vi "Initialize Protection Frames Incoming.vi"(8 "error in (no error)":errorcluster, 10 "Frames":T2[](array[typedef]) {"Protection Configurations"."CRC Channels"."Data Type" items=["Signed", "Unsigned", "IEEE Float"]}, 11 "PCL (usec)":u32) -> (0 "error out":errorcluster, 1 "Frame Values":T1, 2 "RT Frames":T9[](array[typedef]) {"Protection Configurations"."CRC Channels"."Data Type" items=["Signed", "Unsigned", "IEEE Float"]})   [LabVIEW 2023, in "Protection and Counter Support Engine.lvlib"]
uses:
  Protection and Counter Support Engine.lvlib
  Types/RT Frame Settings.ctl
  Shared/Types/Exported Frame Type.ctl
  Types/RT Protection Configuration.ctl
  Shared/Types/Protection Type.ctl
  Shared/Types/XNET Signal Configuration.ctl
  Shared/Types/Exported Counter Settings.ctl
  Shared/Types/Exported Event Trigger Type.ctl
  Shared/Types/Exported Frame Settings.ctl
  Shared/Types/Exported Protection Settings.ctl
  Types/RT Frame Incoming Values.ctl
  <vilib>/xnet/xnet.llb/XNET Create Session (Conversion).vi
  Shared/Protection and Counter Support Shared.lvlib
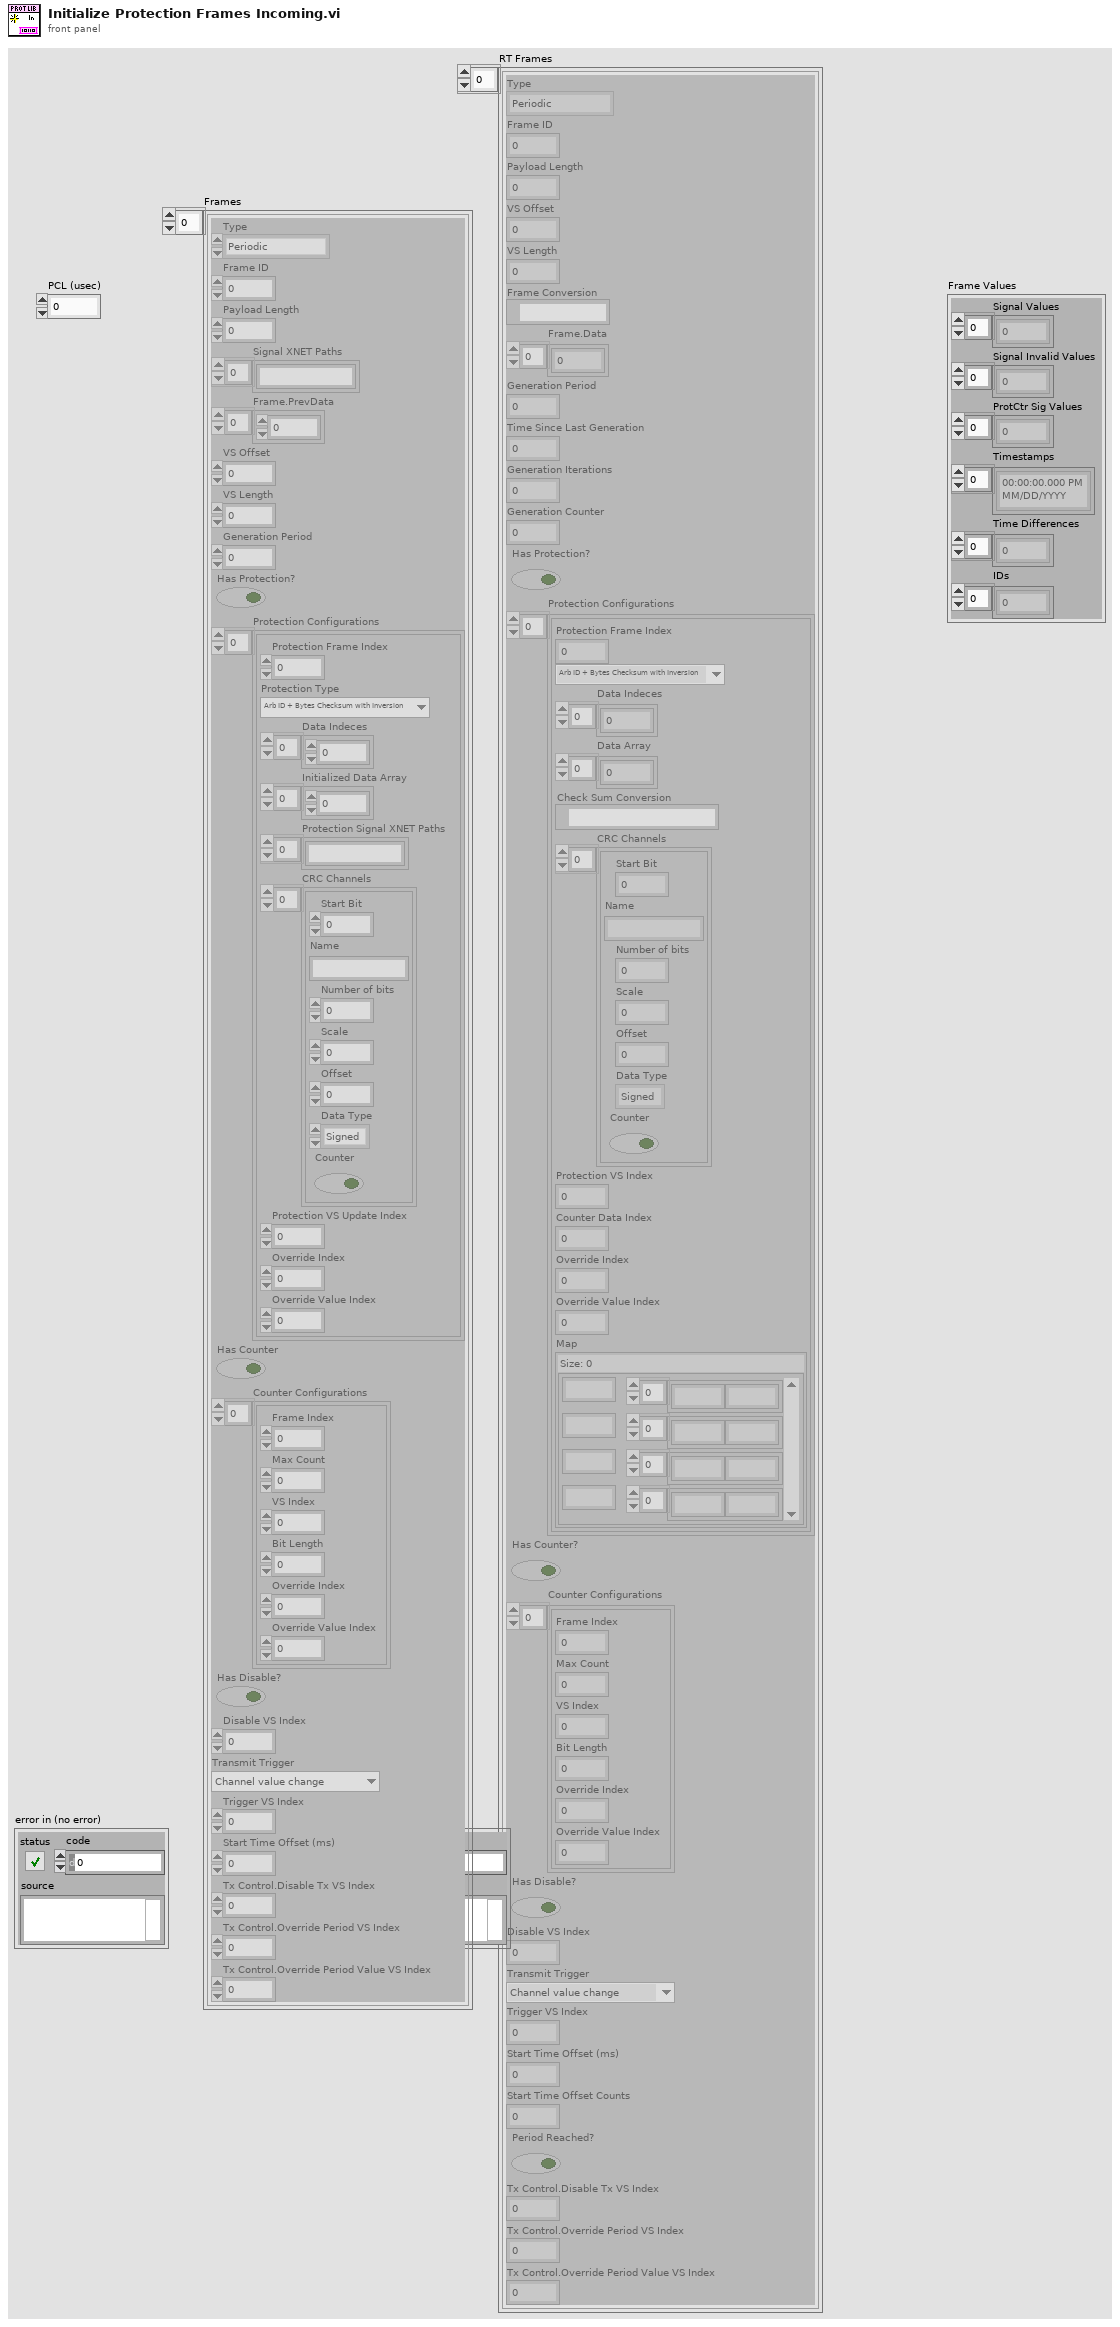
[diagram p1: front panel]
types:
  T1 = typedef "Protection and Counter Support Engine.lvlib/RT Frame Incoming Values.ctl" = cluster{"Signal Values":dbl[], "Signal Invalid Values":dbl[], "ProtCtr Sig Values":dbl[], "Timestamps":timestamp[], "Time Differences":dbl[], "IDs":u32[]}
  T2 = typedef "Protection and Counter Support Shared.lvlib/Exported Frame Settings.ctl" = cluster{"Type":T3, "Frame ID":u32, "Payload Length":u32, "Signal XNET Paths":string[], "Frame.PrevData":dbl[], "VS Offset":i32, "VS Length":i32, "Generation Period":u32, "Has Protection?":bool, "Protection Configurations":T4[], "Has Counter":bool, "Counter Configurations":T7[], "Has Disable?":bool, "Disable VS Index":i32, "Transmit Trigger":T8, "Trigger VS Index":i32, "Start Time Offset (ms)":u32, "Tx Control.Disable Tx VS Index":i32, "Tx Control.Override Period VS Index":i32, "Tx Control.Override Period Value VS Index":i32}
  T3 = typedef "Protection and Counter Support Shared.lvlib/Exported Frame Type.ctl" = enum16{"Periodic", "Event", "Periodic/Event"}
  T4 = typedef "Protection and Counter Support Shared.lvlib/Exported Protection Settings.ctl" = cluster{"Protection Frame Index":i32, "Protection Type":T5, "Data Indeces":i32[], "Initialized Data Array":dbl[], "Protection Signal XNET Paths":string[], "CRC Channels":T6[], "Protection VS Update Index":i32, "Override Index":i32, "Override Value Index":i32}
  T5 = typedef "Protection and Counter Support Shared.lvlib/Protection Type.ctl" = enum16{"Arb ID + Bytes Checksum with Inversion", "Arb ID + Bytes CRC with Inversion", "Reversed Raw Signal Checksum with Inversion", "Concatenated Two's Compliment", "LP_CRC8", "LP_Checksum", "LP_CRC8_MRS"}
  T6 = typedef "Protection and Counter Support Shared.lvlib/XNET Signal Configuration.ctl" = cluster{"Start Bit":i32, "Name":string, "Number of bits":i32, "Scale":dbl, "Offset":dbl, "Data Type":u32, "Counter":bool}
  T7 = typedef "Protection and Counter Support Shared.lvlib/Exported Counter Settings.ctl" = cluster{"Frame Index":i32, "Max Count":dbl, "VS Index":i32, "Bit Length":i64, "Override Index":i32, "Override Value Index":i32}
  T8 = typedef "Protection and Counter Support Shared.lvlib/Exported Event Trigger Type.ctl" = enum16{"Channel value change", "Trigger channel (not zero)", "Channel value change or trigger channel (not zero)", "Trigger channel (any value change)", "Channel value change or trigger channel (any value change)"}
  T9 = typedef "Protection and Counter Support Engine.lvlib/RT Frame Settings.ctl" = cluster{"Type":T3, "Frame ID":u32, "Payload Length":u32, "VS Offset":i32, "VS Length":i32, "Frame Conversion":refnum<k21>, "Frame.Data":dbl[], "Generation Period":u32, "Time Since Last Generation":u32, "Generation Iterations":u32, "Generation Counter":u32, "Has Protection?":bool, "Protection Configurations":T10[], "Has Counter?":bool, "Counter Configurations":T7[], "Has Disable?":bool, "Disable VS Index":i32, "Transmit Trigger":T8, "Trigger VS Index":i32, "Start Time Offset (ms)":u32, "Start Time Offset Counts":u32, "Period Reached?":bool, "Tx Control.Disable Tx VS Index":i32, "Tx Control.Override Period VS Index":i32, "Tx Control.Override Period Value VS Index":i32}
  T10 = typedef "Protection and Counter Support Engine.lvlib/RT Protection Configuration.ctl" = cluster{"Protection Frame Index":i32, "Protection Type":T5, "Data Indeces":i32[], "Data Array":dbl[], "Check Sum Conversion":refnum<k21>, "CRC Channels":T6[], "Protection VS Index":i32, "Counter Data Index":i32, "Override Index":i32, "Override Value Index":i32, "Map":map{i32, u8[]}}
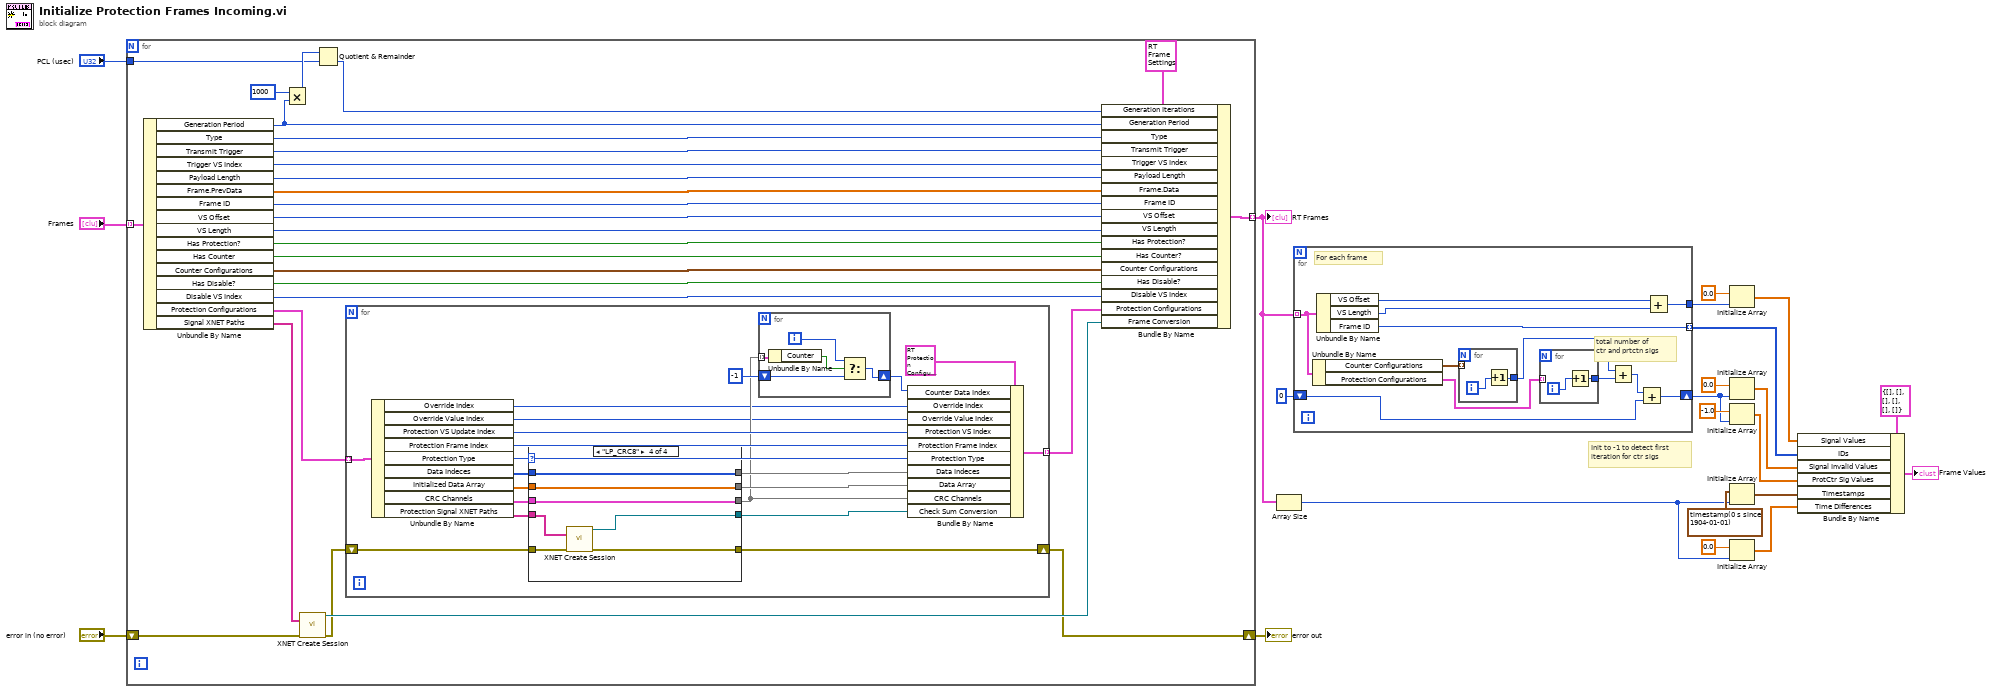
[diagram p0: block diagram]
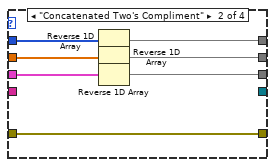
[diagram p3: hidden frame]
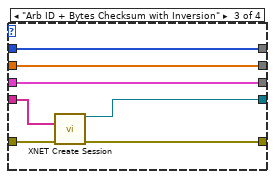
[diagram p4: hidden frame]
diagram:
  # "Init to -1 to detect first \niteration for ctr sigs"
  n1 = for {
    shift-right: [w35] -> w20
    shift-left: "error in (no error)" -> [w48]
    tunnel: "Frames" -> [w50] mode=indexing
    tunnel: [w34] -> w1 mode=indexing
    tunnel: "PCL (usec)" -> [w29]
    n2 = Unbundle By Name(w50) -> ("Generation Period"=w28:u32, "Type"=w23:T3, "Transmit Trigger"=w24:T8, "Trigger VS Index"=w25:i32, "Payload Length"=w26:u32, "Frame.PrevData"=w32:dbl[], "Frame ID"=w46:u32, "VS Offset"=w45:i32, "VS Length"=w44:i32, "Has Protection?"=w43:bool, "Has Counter"=w42:bool, "Counter Configurations"=w41:T7[], "Has Disable?"=w40:bool, "Disable VS Index"=w39:i32, "Protection Configurations"=w38:T4[], "Signal XNET Paths"=w49:string[])
    n3 = Multiply(x=u32 1000, y=w28) -> (x*y=w30:u32)
    n4 = call-poly <vilib>:"XNET Create Session.vi"("signal list"=w49, "error in (no error)"=w48) -> ("session out"=w47:refnum<k21>, "error out"=w36:errorcluster)  [unwired: 12 out]
    n5 = Quotient & Remainder(x=w30, y=w29) -> (floor(x/y)=w27:u32)  [unwired: 1 out]
    n6 = for {
      tunnel: w38 -> [w70] mode=indexing
      tunnel: [w65] -> w37 mode=indexing
      shift-right: [w63] -> w35
      shift-left: w36 -> [w64]
      n7 = Unbundle By Name(w70) -> ("Override Index"=w52:i32, "Override Value Index"=w51:i32, "Protection VS Update Index"=w54:i32, "Protection Frame Index"=w68:i32, "Protection Type"=w60:T5, "Data Indeces"=w55:i32[], "Initialized Data Array"=w57:dbl[], "CRC Channels"=w59:T6[], "Protection Signal XNET Paths"=w67:string[])
      n8 = case shown="\"LP_CRC8\"" w60 {
        tunnel: w67 -> [_ _ w88 w95]
        tunnel: [_ _ w87 w94] -> w66
        tunnel: w64 -> [w74 w81 w86 w93]
        tunnel: [w74 w81 w85 w92] -> w63
        tunnel: [w73 w77 w84 w91] -> w53
        tunnel: w59 -> [w73 w80 w84 w91]
        tunnel: [w72 w76 w83 w90] -> w58
        tunnel: w57 -> [w72 w79 w83 w90]
        tunnel: [w71 w75 w82 w89] -> w56
        tunnel: w55 -> [w71 w78 w82 w89]
        frame Default {
        }
        frame "Concatenated Two's Compliment" {
          n9 = Reverse 1D Array(array=w78) -> (reversed array=w75:i32[])
          n10 = Reverse 1D Array(array=w79) -> (reversed array=w76:dbl[])
          n11 = Reverse 1D Array(array=w80) -> (reversed array=w77:T6[])
        }
        frame "Arb ID + Bytes Checksum with Inversion" {
          n12 = call-poly <vilib>:"XNET Create Session.vi"("signal list"=w88, "error in (no error)"=w86) -> ("session out"=w87:refnum<k21>, "error out"=w85:errorcluster)  [unwired: 12 out]
        }
        frame "LP_CRC8" {
          n13 = call-poly <vilib>:"XNET Create Session.vi"("signal list"=w95, "error in (no error)"=w93) -> ("session out"=w94:refnum<k21>, "error out"=w92:errorcluster)  [unwired: 12 out]
        }
      }
      n14 = for {
        tunnel: w53 -> [w100] mode=indexing
        shift-right: [w96] -> w61
        shift-left: -1 -> [w98]
        i -> [w97]
        n15 = Unbundle By Name(w100) -> ("Counter"=w99:bool)
        n16 = Select(t=w97, s=w99, f=w98) -> (s? t:f=w96:i32)
      }
      n17 = Bundle By Name(cluster=T10 {"Protection Frame Index"=0, "Protection Type"=enum."Arb ID + Bytes Checksum with Inversion", "Data Indeces"=[], "Data Array"=[], "Check Sum Conversion"="", "CRC Channels"=[], "Protection VS Index"=0, "Counter Data Index"=0, "Override Index"=0, "Override Value Index"=0, "Map"={}} ("Cluster"), "Counter Data Index"=w61, "Override Index"=w52, "Override Value Index"=w51, "Protection VS Index"=w54, "Protection Frame Index"=w68, "Protection Type"=w60, "Data Indeces"=w56, "Data Array"=w58, "CRC Channels"=w53, "Check Sum Conversion"=w66) -> (w65:T10)
    }
    n18 = Bundle By Name(cluster=T9 {"Type"=enum."Periodic", "Frame ID"=0, "Payload Length"=0, "VS Offset"=0, "VS Length"=0, "Frame Conversion"="", "Frame.Data"=[], "Generation Period"=0, "Time Since Last Generation"=0, "Generation Iterations"=0, "Generation Counter"=0, "Has Protection?"=FALSE, "Protection Configurations"=[], "Has Counter?"=FALSE, "Counter Configurations"=[], "Has Disable?"=FALSE, "Disable VS Index"=0, "Transmit Trigger"=enum."Channel value change", "Trigger VS Index"=0, "Start Time Offset (ms)"=0, "Start Time Offset Counts"=0, "Period Reached?"=FALSE, "Tx Control.Disable Tx VS Index"=0, "Tx Control.Override Period VS Index"=0, "Tx Control.Override Period Value VS Index"=0} ("Frame Settings"), "Generation Iterations"=w27, "Generation Period"=w28, "Type"=w23, "Transmit Trigger"=w24, "Trigger VS Index"=w25, "Payload Length"=w26, "Frame.Data"=w32, "Frame ID"=w46, "VS Offset"=w45, "VS Length"=w44, "Has Protection?"=w43, "Has Counter?"=w42, "Counter Configurations"=w41, "Has Disable?"=w40, "Disable VS Index"=w39, "Protection Configurations"=w37, "Frame Conversion"=w47) -> (w34:T9)
  }
  "RT Frames" <- w1
  "error out" <- w20
  n19 = Array Size(array=w1) -> (size(s)=w6:i32)
  n20 = for {
    tunnel: w1 -> [w108] mode=indexing
    tunnel: [w112] -> w18 mode=indexing
    tunnel: [w109] -> w16
    shift-right: [w102] -> w12
    shift-left: 0 -> [w101]
    # "total number of\nctr and prtctn sigs"
    # "For each frame"
    n21 = Unbundle By Name(w108) -> ("Counter Configurations"=w107:T7[], "Protection Configurations"=w106:T10[])
    n22 = Unbundle By Name(w108) -> ("VS Offset"=w111:i32, "VS Length"=w110:i32, "Frame ID"=w112:u32)
    n23 = for {
      tunnel: w107 -> [_] mode=indexing
      tunnel: [w115] -> w105
      i -> [w116]
      n24 = Increment(x=w116) -> (x+1=w115:i32)
    }
    n25 = for {
      tunnel: [w113] -> w104
      tunnel: w106 -> [_] mode=indexing
      i -> [w114]
      n26 = Increment(x=w114) -> (x+1=w113:i32)
    }
    n27 = Add(x=w105, y=w104) -> (x+y=w103:i32)
    n28 = Add(x=w103, y=w101) -> (x+y=w102:i32)
    n29 = Add(x=w111, y=w110) -> (x+y=w109:i32)
  }
  n30 = Initialize Array(0.0, w16) -> (w15:dbl[])
  n31 = Initialize Array(0.0, w12) -> (w10:dbl[])
  n32 = Initialize Array(-1.0, w12) -> (w11:dbl[])
  n33 = Initialize Array(timestamp(0 s since 1904-01-01) ("Time Stamp"), w6) -> (w7:timestamp[])
  n34 = Initialize Array(0.0, w6) -> (w4:dbl[])
  n35 = Bundle By Name(cluster=T1 {"Signal Values"=[], "Signal Invalid Values"=[], "ProtCtr Sig Values"=[], "Timestamps"=[], "Time Differences"=[], "IDs"=[]} ("Incoming Values"), "Signal Values"=w15, "IDs"=w18, "Signal Invalid Values"=w10, "ProtCtr Sig Values"=w11, "Timestamps"=w7, "Time Differences"=w4) -> (→"Frame Values":T1)
